vi "Data To API String Arguments.vi"(7 "reference cluster data":variant, 9 "error in (no error)":errorcluster, 11 "data":variant) -> (1 "error out":errorcluster, 3 "String":string)   [LabVIEW 2017, in "API String Arguments Support.lvlib"]
uses:
  API String Arguments Support.lvlib
  <userlib>/_NEVSTOP/Communicable State Machine(CSM)/_Support/KeyWords.vi
  <userlib>/_OpenG.lib/array/array.llb/Filter 1D Array with Scalar (String)__ogtk.vi
  <vilib>/Utility/Data Type/NI_Data Type.lvlib
  <userlib>/_NEVSTOP/Communicable State Machine(CSM)/Communicable State Machine.lvlib
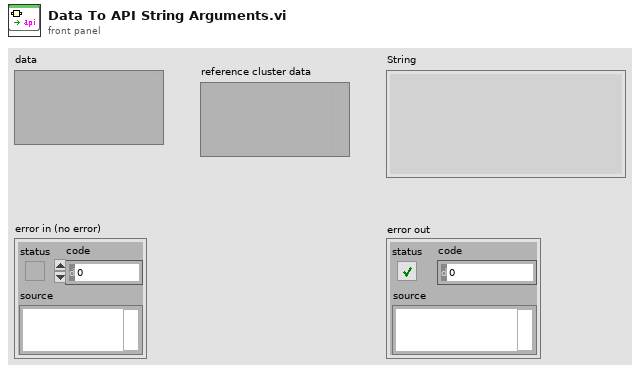
[diagram p1: front panel]
types:
  T1 = typedef "NI_Data Type.lvlib/Data Type.ctl" = enum8{"Invalid Type", "Void", "I8", "I16", "I32", "I64", "U8", "U16", "U32", "U64", "Single Float", "Double Float", "Extended Float", "Single Complex", "Double Complex", "Extended Complex", "Enum U8", "Enum U16", "Enum U32", "Enum U64", "Single Float With Unit", "Double Float With Unit", "Extended Float With Unit", "Single Complex with Unit", "Double Complex with Unit", "Extended Complex with Unit", "Boolean", "String", "Path", "Picture", "Tag", "Array", "Cluster", "Variant", "LV Variant", "Waveform", "Timestamp", "Digital Waveform", "Digital Data", "ExpressData", "Refnum", "External Data", "VI", "Poly VI", "LabVIEW Class Instance", "Fixed Point"}
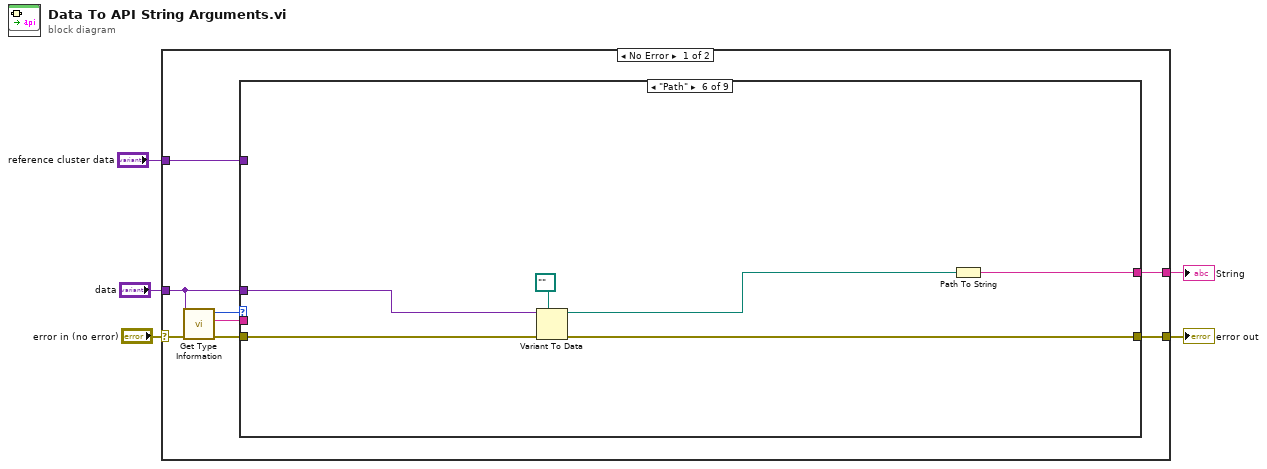
[diagram p0: block diagram]
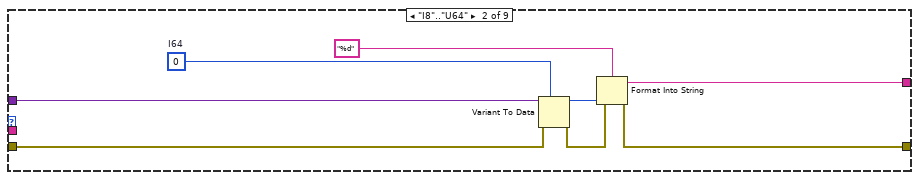
[diagram p3: hidden frame]
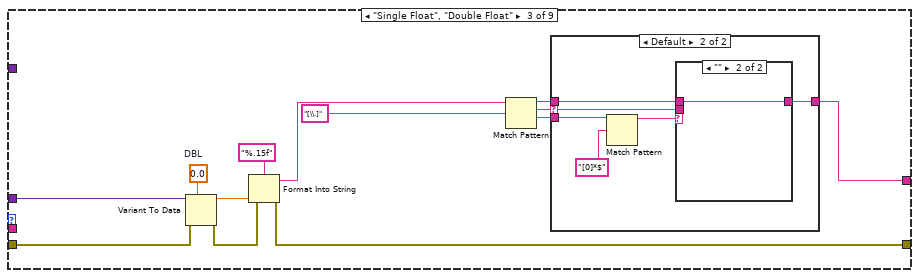
[diagram p4: hidden frame]
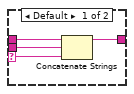
[diagram p6: hidden frame]
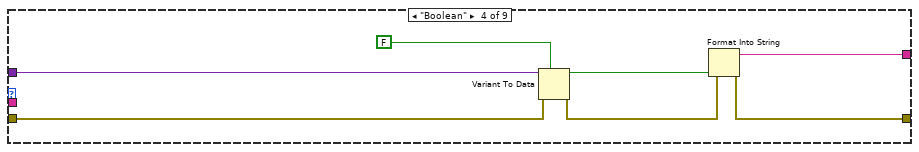
[diagram p7: hidden frame]
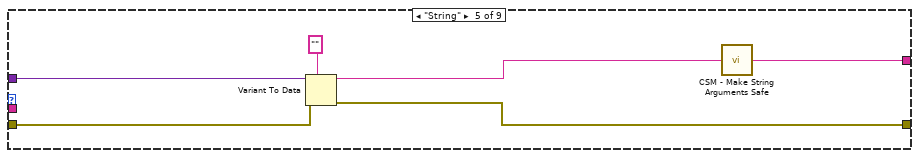
[diagram p8: hidden frame]
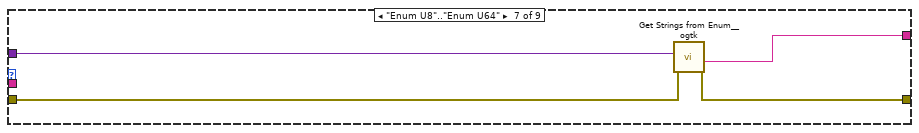
[diagram p9: hidden frame]
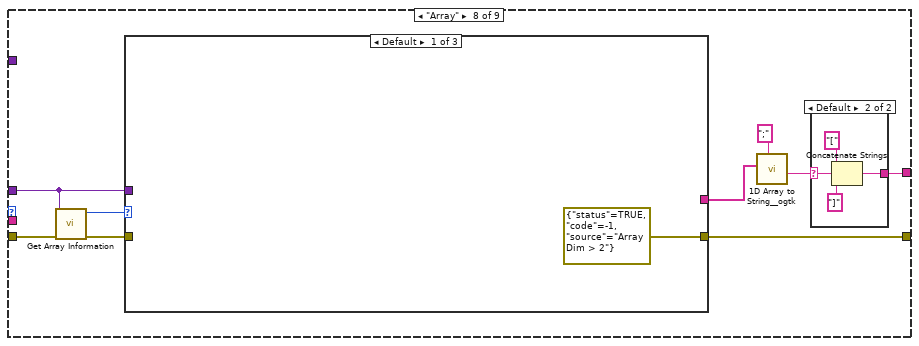
[diagram p10: hidden frame]
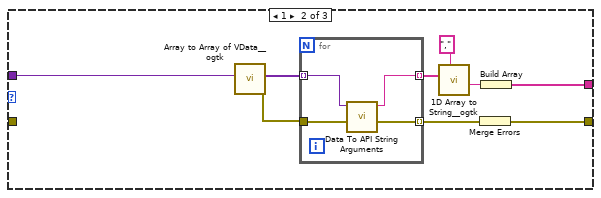
[diagram p11: hidden frame]
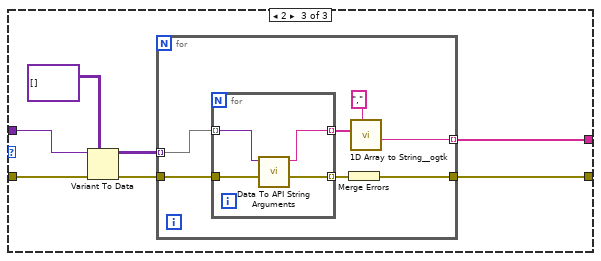
[diagram p12: hidden frame]
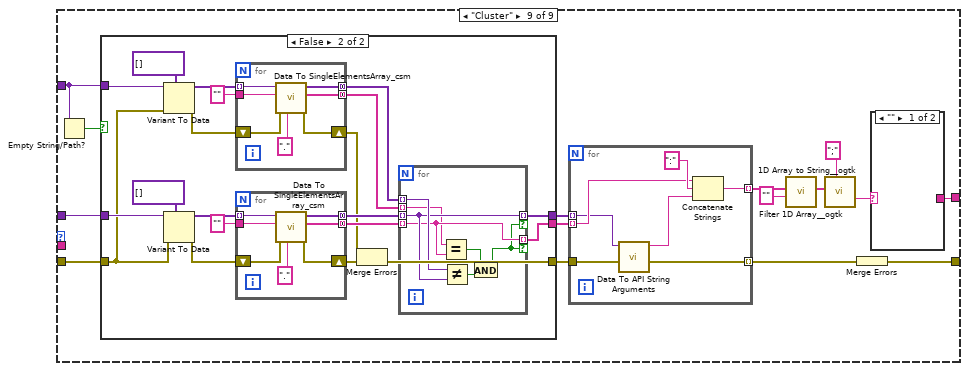
[diagram p14: hidden frame]
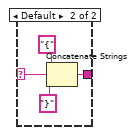
[diagram p15: hidden frame]
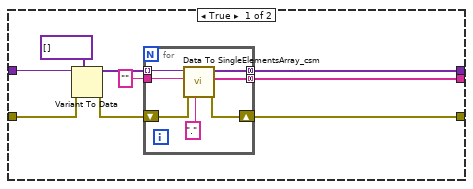
[diagram p16: hidden frame]
diagram:
  n1 = case shown="No Error" "error in (no error)" {
    selector: "error in (no error)" -> [w7 w199]
    tunnel: [w11 _] -> w5
    tunnel: "data" -> [w10 _]
    tunnel: [w8 w199] -> w3
    tunnel: "reference cluster data" -> [w6 _]
    frame No Error {
      n2 = call <vilib>:"Get Type Information.vi"("error in (no error)"=w7, "Variant"=w10) -> ("error out"=w9:errorcluster, "Name"=w12:string, "Type"=w13:T1)  [unwired: 5 in, 2 out]
      n3 = case shown="\"Path\"" w13 {
        tunnel: w12 -> [_ _ _ _ _ _ _ _ _]
        tunnel: [_ w18 w23 w52 w55 w61 w69 w79 w130] -> w11
        tunnel: w10 -> [_ w22 w35 w54 w60 w66 w70 w77 w122]
        tunnel: w9 -> [w14 w17 w32 w51 w58 w64 w68 w78 w121]
        tunnel: [w14 w15 w30 w49 w57 w63 w67 w75 w128] -> w8
        tunnel: w6 -> [_ _ _ _ _ _ _ _ w116]
        frame "Invalid Type", "Void", Default {
        }
        frame "I8".."U64" {
          w21 = i64 0  # I64
          n4 = Variant To Data(error in=w17, type=w21, Variant=w22) -> (data=w20:i64, error out=w16:errorcluster)
          n5 = Format Into String(format string="%d", error in=w16, w20) -> (resulting string=w18:string, error out=w15:errorcluster)  [unwired: 1 in]
        }
        frame "Single Float", "Double Float" {
          w29 = 0.0  # DBL
          n6 = Variant To Data(error in=w32, type=w29, Variant=w35) -> (data=w34:dbl, error out=w31:errorcluster)
          n7 = Format Into String(format string="%.15f", error in=w31, w34) -> (resulting string=w28:string, error out=w30:errorcluster)  [unwired: 1 in]
          n8 = Match Pattern(string=w28, regular expression="[\\.]") -> (before substring=w25:string, match substring=w24:string, after substring=w26:string)  [unwired: 1 in, 1 out]
          n9 = case shown="Default" w24 {
            selector: w24 -> [_ w39]
            tunnel: w26 -> [_ w42]
            tunnel: w25 -> [w36 w40]
            tunnel: [w36 w37] -> w23
            frame "" {
            }
            frame Default {
              n10 = Match Pattern(string=w42, regular expression="[0]*$") -> (before substring=w38:string)  [unwired: 1 in, 3 out]
              n11 = case shown="\"\"" w38 {
                selector: w38 -> [w44 _]
                tunnel: w40 -> [w46 w47]
                tunnel: w39 -> [w45 _]
                tunnel: [w43 w47] -> w37
                frame Default {
                  n12 = Concatenate Strings(w46, w45, w44) -> (w43:string)
                }
                frame "" {
                }
              }
            }
          }
        }
        frame "Boolean" {
          n13 = Variant To Data(error in=w51, type=FALSE, Variant=w54) -> (data=w53:bool, error out=w50:errorcluster)
          n14 = Format Into String(error in=w50, w53) -> (resulting string=w52:string, error out=w49:errorcluster)  [unwired: 2 in]
        }
        frame "String" {
          n15 = Variant To Data(error in=w58, type="", Variant=w60) -> (data=w59:string, error out=w57:errorcluster)
          n16 = call <userlib>:"CSM - Make String Arguments Safe.vi"("Argurment String"=w59) -> ("Safe Argurment String"=w55:string)  [unwired: 8 in]
        }
        frame "Path" {
          n17 = Variant To Data(error in=w64, type=path "", Variant=w66) -> (data=w65:path, error out=w63:errorcluster)
          n18 = Path To String(path=w65) -> (string=w61:string)
        }
        frame "Enum U8".."Enum U64" {
          n19 = call <userlib>:"Get Strings from Enum__ogtk.vi"("error in (no error)"=w68, "Enum"=w70) -> ("error out"=w67:errorcluster, "String Value"=w69:string)  [unwired: 6 in, 2 out]
        }
        frame "Array" {
          n20 = call <vilib>:"Get Array Information.vi"("error in (no error)"=w78, "Variant"=w77) -> ("error out"=w71:errorcluster, "Number of Dimensions"=w76:i32)  [unwired: 6 in, 2 out]
          n21 = case shown="Default" w76 {
            tunnel: [errorcluster {"status"=TRUE, "code"=-1, "source"="Array Dim > 2"} ("error IO") w82 w98] -> w75
            tunnel: [_ w81 w100] -> w73
            tunnel: w77 -> [_ w83 w99]
            tunnel: w71 -> [_ _ w97]
            frame Default {
            }
            frame 1 {
              n22 = call <userlib>:"Array to Array of VData__ogtk.vi"("MultiD Array"=w83) -> ("error out"=w88:errorcluster, "1D Array of Variants"=w89:variant[])  [unwired: 9 in]
              n23 = for {
                tunnel: w89 -> [w93] mode=indexing
                tunnel: w88 -> [w91]
                tunnel: [w92] -> w87 mode=indexing
                tunnel: [w90] -> w86 mode=indexing
                n24 = call "Data To API String Arguments.vi"("error in (no error)"=w91, "data"=w93) -> ("error out"=w92:errorcluster, "String"=w90:string)  [unwired: 8 in]
              }
              n25 = call <userlib>:"1D Array to String__ogtk.vi"("delimiter (Tab)"=",", "Array of Strings"=w86) -> ("delimited string"=w84:string)  [unwired: 9 in]
              n26 = Merge Errors(w87) -> (w82:errorcluster)
              n27 = Build Array(w84) -> (w81:string[])
            }
            frame 2 {
              n28 = Variant To Data(error in=w97, type=variant[][] [], Variant=w99) -> (data=w94:variant[][], error out=w95:errorcluster)
              n29 = for {
                tunnel: [w105] -> w100 mode=indexing
                tunnel: [w104] -> w98
                tunnel: w95 -> [w102]
                tunnel: w94 -> [w101] mode=indexing
                n30 = for {
                  tunnel: w101 -> [w111] mode=indexing
                  tunnel: w102 -> [w109]
                  tunnel: [w110] -> w103 mode=indexing
                  tunnel: [w108] -> w107 mode=indexing
                  n31 = call "Data To API String Arguments.vi"("error in (no error)"=w109, "data"=w111) -> ("error out"=w110:errorcluster, "String"=w108:string)  [unwired: 8 in]
                }
                n32 = Merge Errors(w103) -> (w104:errorcluster)
                n33 = call <userlib>:"1D Array to String__ogtk.vi"("delimiter (Tab)"=",", "Array of Strings"=w107) -> ("delimited string"=w105:string)  [unwired: 9 in]
              }
            }
          }
          n34 = call <userlib>:"1D Array to String__ogtk.vi"("delimiter (Tab)"=";", "Array of Strings"=w73) -> ("delimited string"=w72:string)  [unwired: 9 in]
          n35 = case shown="Default" w72 {
            selector: w72 -> [_ w112]
            tunnel: [_ w115] -> w79
            frame "" {
            }
            frame Default {
              n36 = Concatenate Strings("[" ("string"), w112, "]" ("string")) -> (w115:string)
            }
          }
        }
        frame "Cluster" {
          n37 = Empty String/Path?(string/path=w116) -> (empty?=w117:bool)
          n38 = case shown="False" w117 {
            tunnel: w122 -> [w139 w166]
            tunnel: w121 -> [w138 w160]
            tunnel: [w137 w156] -> w120
            tunnel: [w136 w152] -> w119
            tunnel: [w135 w154] -> w118
            tunnel: w116 -> [_ w161]
            frame True {
              n39 = Variant To Data(error in=w138, type=variant[] [] ("Array"), Variant=w139) -> (data=w141:variant[], error out=w140:errorcluster)
              n40 = for {
                tunnel: [w148] -> w137 mode=concatenating
                tunnel: [w146] -> w135 mode=concatenating
                tunnel: "" ("parentUrl") -> [w145]
                tunnel: w141 -> [w144] mode=indexing
                shift-right: [w147] -> w136
                shift-left: w140 -> [w150]
                n41 = call "Data To SingleElementsArray_csm.vi"("Seperator(/)"=".", "error in (no error)"=w150, "parentUrl"=w145, "Cluster"=w144) -> ("error out"=w147:errorcluster, "Full NameList"=w146:string[], "DataElementArray"=w148:variant[])  [unwired: 5 in]
              }
            }
            frame False {
              n42 = Variant To Data(error in=w160, type=variant[] [] ("Array"), Variant=w161) -> (data=w164:variant[], error out=w165:errorcluster)
              n43 = Variant To Data(error in=w160, type=variant[] [] ("Array"), Variant=w166) -> (data=w168:variant[], error out=w167:errorcluster)
              n44 = for {
                tunnel: [w182] -> w159 mode=concatenating
                tunnel: [w180] -> w158 mode=concatenating
                tunnel: "" ("parentUrl") -> [w179]
                tunnel: w164 -> [w178] mode=indexing
                shift-right: [w181] -> w151
                shift-left: w165 -> [w184]
                n45 = call "Data To SingleElementsArray_csm.vi"("Seperator(/)"=".", "error in (no error)"=w184, "parentUrl"=w179, "Cluster"=w178) -> ("error out"=w181:errorcluster, "Full NameList"=w180:string[], "DataElementArray"=w182:variant[])  [unwired: 5 in]
              }
              n46 = for {
                tunnel: [w189] -> w157 mode=concatenating
                tunnel: [w187] -> w155 mode=concatenating
                tunnel: "" ("parentUrl") -> [w186]
                tunnel: w168 -> [w185] mode=indexing
                shift-right: [w188] -> w153
                shift-left: w167 -> [w191]
                n47 = call "Data To SingleElementsArray_csm.vi"("Seperator(/)"=".", "error in (no error)"=w191, "parentUrl"=w186, "Cluster"=w185) -> ("error out"=w188:errorcluster, "Full NameList"=w187:string[], "DataElementArray"=w189:variant[])  [unwired: 5 in]
              }
              n48 = Merge Errors(w151, w153) -> (w152:errorcluster)
              n49 = for {
                tunnel: w159 -> [w177] mode=indexing
                tunnel: w157 -> [w176] mode=indexing
                tunnel: w158 -> [w173] mode=indexing
                tunnel: w155 -> [w174] mode=indexing
                tunnel: [w176] -> w156 mode=indexing if=w172
                tunnel: [w174] -> w154 mode=indexing if=w172
                n50 = Equal?(x=w173, y=w174) -> (x = y?=w171:bool)
                n51 = Not Equal?(x=w177, y=w176) -> (x != y?=w175:bool)
                n52 = And(x=w171, y=w175) -> (x .and. y?=w172:bool)
              }
            }
          }
          n53 = for {
            tunnel: [w192] -> w129 mode=indexing
            tunnel: [w198] -> w125 mode=indexing
            tunnel: w120 -> [w195] mode=indexing
            tunnel: w119 -> [w193]
            tunnel: w118 -> [w196] mode=indexing
            n54 = call "Data To API String Arguments.vi"("error in (no error)"=w193, "data"=w195) -> ("error out"=w192:errorcluster, "String"=w194:string)  [unwired: 8 in]
            n55 = Concatenate Strings(w196, ":" ("string"), w194) -> (w198:string)
          }
          n56 = call-poly <userlib>:"Filter 1D Array__ogtk.vi"("items to filter"="" ("String"), "array"=w125) -> ("filtered array"=w124:string[])  [unwired: 4 in, 1 out]
          n57 = call <userlib>:"1D Array to String__ogtk.vi"("delimiter (Tab)"=";", "Array of Strings"=w124) -> ("delimited string"=w126:string)  [unwired: 9 in]
          n58 = Merge Errors(w129) -> (w128:errorcluster)
          n59 = case shown="\"\"" w126 {
            selector: w126 -> [_ w131]
            tunnel: [_ w134] -> w130
            frame "" {
            }
            frame Default {
              n60 = Concatenate Strings("{" ("string"), w131, "}" ("string")) -> (w134:string)
            }
          }
        }
      }
    }
    frame Error {
    }
  }
  "String" <- w5
  "error out" <- w3
